vi "Gui_SetupData.vi"(8 "error in (no error)":errorcluster, 11 "Variant":variant) -> (0 "error out":errorcluster caption="sortie d'erreur", 3 "Variant out":variant)   [LabVIEW 2018]
doc: "This VI setup the parameters for the data acquisition.\n\n1. Init the controls with the previous values.\n2. Wait for the user events, CTRL-Z is disabled.\n3. If Acquisition Duration, Record Length or Sample Rate vaues are changed, update the other controls accordingly.\n4. Limit the Record Length value to 32000000, as this is the max memory size of the board."
uses:
  controls/DATA_Inputs.ctl
  controls/SEQUENCE_Inputs.ctl
  controls/EXCIT_Inputs.ctl
  controls/TIMING_Inputs.ctl
  controls/PROCESSING_Inputs.ctl
  controls/TRAPPING_Inputs.ctl
panel:
  in  "CANCEL":bool
  in  "Vertical Range (pk-pk)":dbl(ring)=10.0 caption="Sample Rate" items=["0.2"=0.2, "0.4"=0.4, "1"=1.0, "2"=2.0, "4"=4.0, "10"=10.0]
  in  "OK":bool
  out "Number Of Acquisitions":i16
  out "DATA Inputs":T1={"Record Length"=100000, "Sample Rate"=10000000.0, "Data Type"=0, "Vertical Range"=10.0, "Acquisition Duration"=100000.0} {"Vertical Range" items=["0.2"=0.2, "0.4"=0.4, "1"=1.0, "2"=2.0, "4"=4.0, "10"=10.0]; "Data Type" items=["I16", "DBL"]; "Sample Rate" items=["1 MHz"=1000000.0, "2 MHz"=2000000.0, "5 MHz"=5000000.0, "10 MHz"=10000000.0, "20 MHz"=20000000.0, "25 MHz"=25000000.0, "50 MHz"=50000000.0, "100 MHz"=100000000.0]}
  in  "Sample Rate":dbl(ring)=10000000.0 items=["1 MHz"=1000000.0, "2 MHz"=2000000.0, "5 MHz"=5000000.0, "10 MHz"=10000000.0, "20 MHz"=20000000.0, "25 MHz"=25000000.0, "50 MHz"=50000000.0, "100 MHz"=100000000.0]
  in  "Acquisition Duration (ms)":dbl
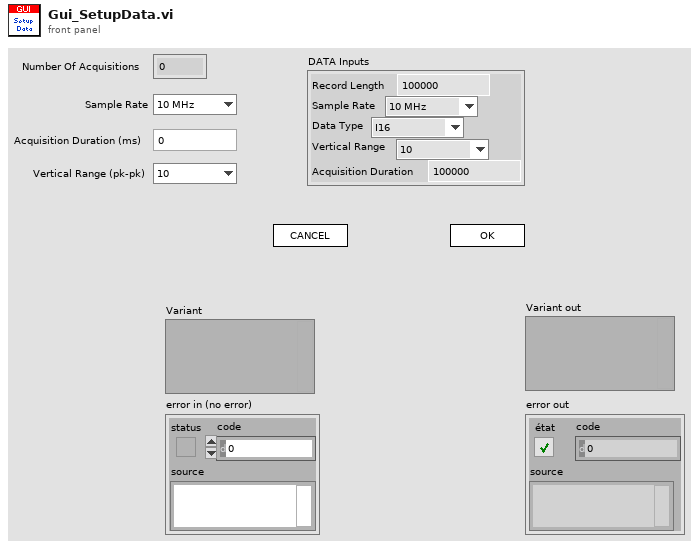
[diagram p1: front panel]
types:
  T1 = typedef "DATA_Inputs.ctl" = cluster{"Record Length":i32, "Sample Rate":dbl, "Data Type":u8, "Vertical Range":dbl, "Acquisition Duration":dbl}
  T2 = typedef "SEQUENCE_Inputs.ctl" = cluster{"EXCIT Inputs":T3, "DATA Inputs":T1, "TIMING Inputs":T4, "PROCESSING Inputs":T5, "TRAPPING Inputs":T6}
  T3 = typedef "EXCIT_Inputs.ctl" = cluster{"Number of Excitations":i32, "Script Text":string, "Table of Waveforms":string[]}
  T4 = typedef "TIMING_Inputs.ctl" = cluster{"Number of Acquisitions ":i16, "Number of Accumulations":i16, "Table of Waveforms":string[], "Script Text":string}
  T5 = typedef "PROCESSING_Inputs.ctl" = cluster{"Reference Mass":dbl, "Cyclotron Freq":dbl, "Magnetron Freq":dbl}
  T6 = typedef "TRAPPING_Inputs.ctl" = cluster{"Number of Channels":i32, "Init Values":dbl[], "Opening Values":dbl[], "Trapping Values":dbl[], "Emptying Values":dbl[], "Adiabatic ON":bool, "Adiabatic Duration":i32, "Adiabatic Waveforms":string[], "Ions Refill ON":bool, "Number of Ions Refills":i32, "Trapping Delay":dbl, "Trapping Duration":dbl}
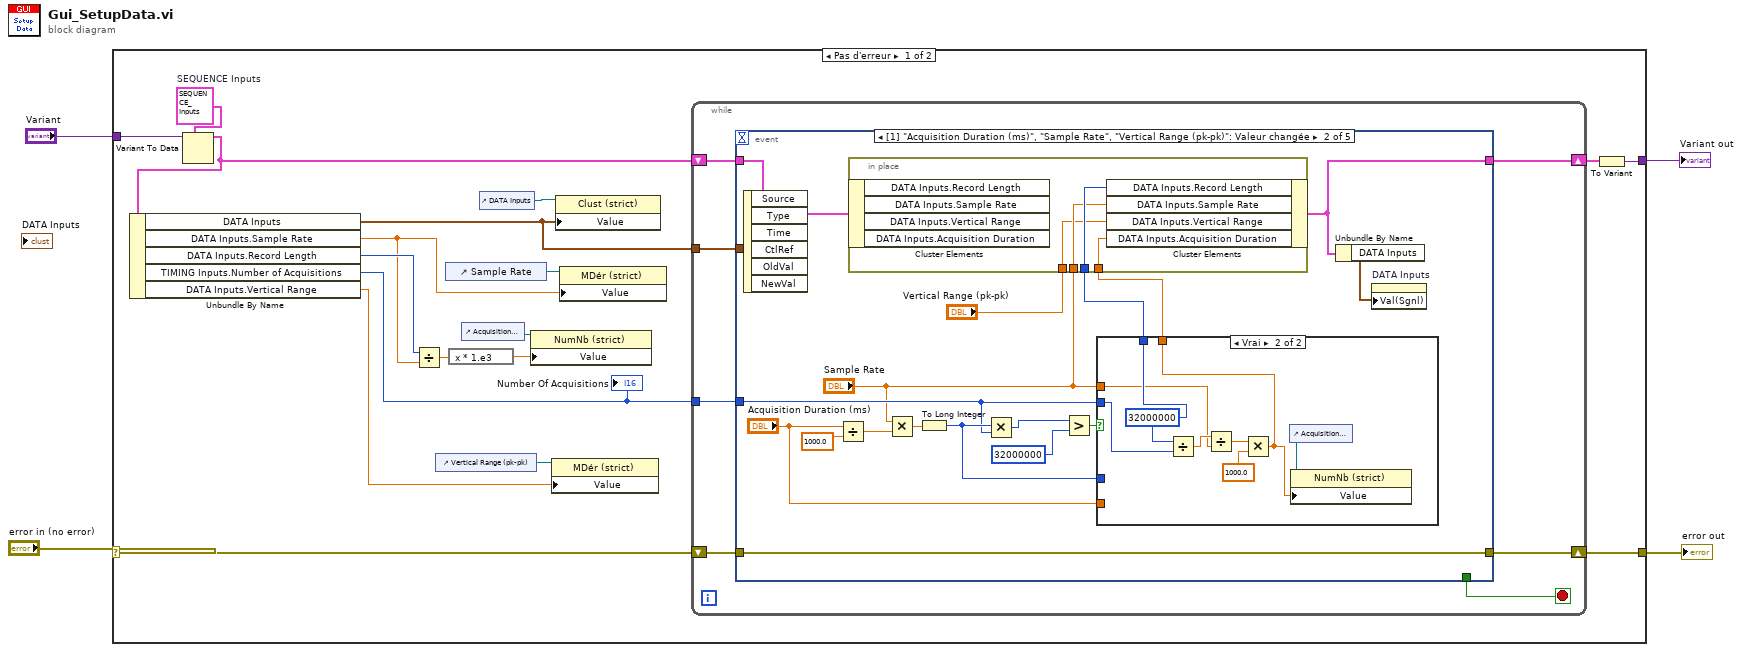
[diagram p0: block diagram]
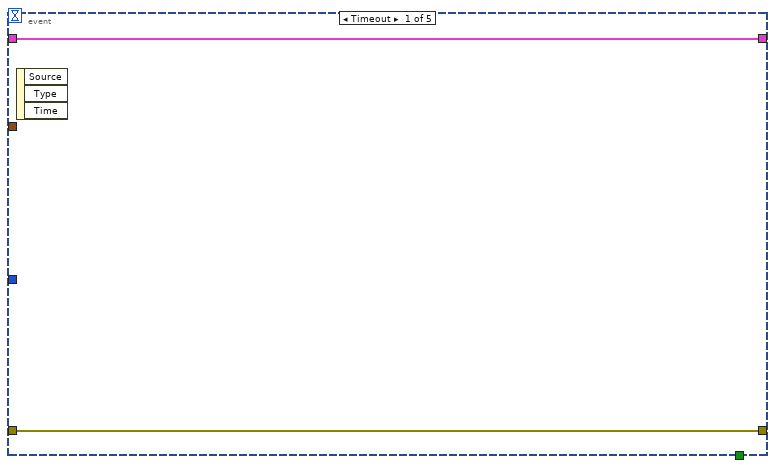
[diagram p2: hidden frame]
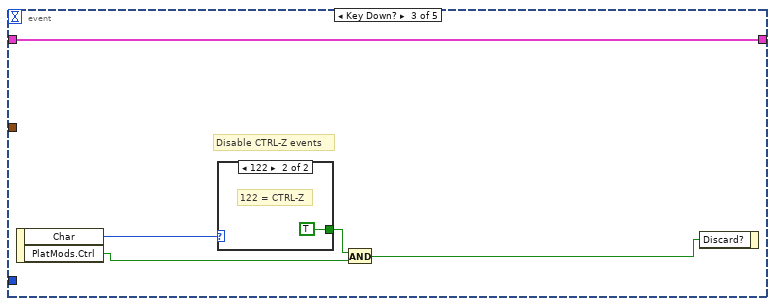
[diagram p4: hidden frame]
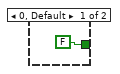
[diagram p5: hidden frame]
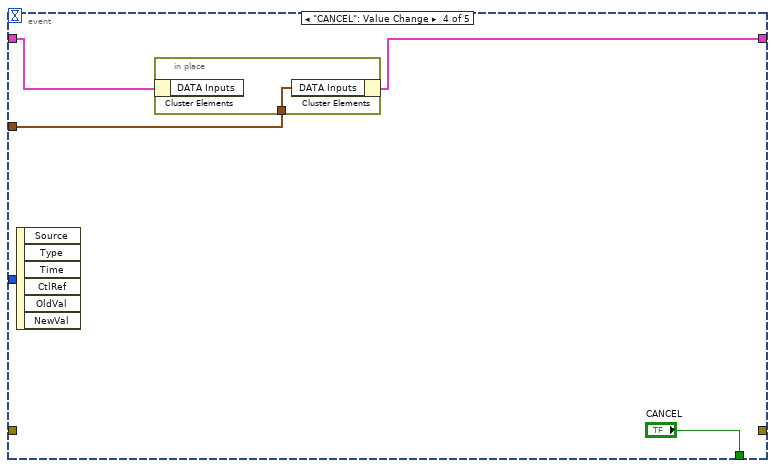
[diagram p6: hidden frame]
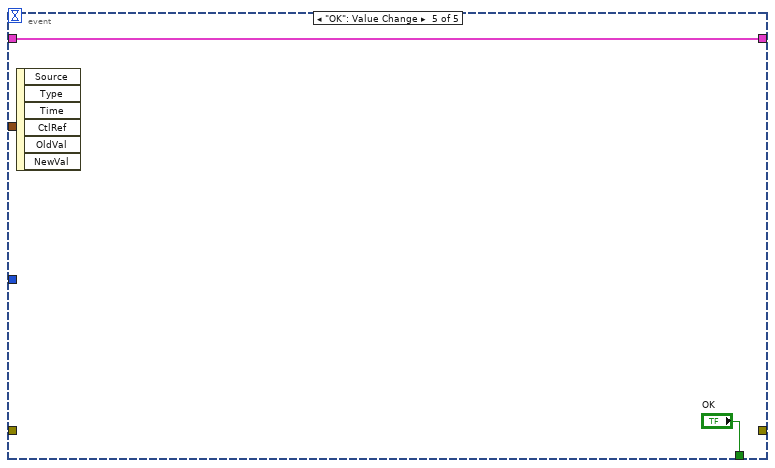
[diagram p7: hidden frame]
diagram:
  n1 = case shown="Pas d'erreur" "error in (no error)" {
    selector: "error in (no error)" -> [w22 w78]
    tunnel: [w21 w78] -> w3
    tunnel: "Variant" -> [w19 w77]
    tunnel: [w10 w77] -> w1
    frame No Error {
      w20 = T2 {"EXCIT Inputs"={"Number of Excitations"=1, "Script Text"="", "Table of Waveforms"=[]}, "DATA Inputs"={"Record Length"=8192, "Sample Rate"=4.0, "Data Type"=0, "Vertical Range"=0.0, "Acquisition Duration"=100000.0}, "TIMING Inputs"={"Number of Acquisitions "=1, "Number of Accumulations"=1, "Table of Waveforms"=[], "Script Text"=""}, "PROCESSING Inputs"={"Reference Mass"=300.0939, "Cyclotron Freq"=255.727, "Magnetron Freq"=0.001}, "TRAPPING Inputs"={"Number of Channels"=4, "Init Values"=[2.0, 5.0, 5.0, 2.0], "Opening Values"=[0.0, 0.0, 0.0, 0.0], "Trapping Values"=[2.0, 5.0, 5.0, 2.0], "Emptying Values"=[-5.0, -5.0, -5.0, -5.0], "Adiabatic ON"=FALSE, "Adiabatic Duration"=0, "Adiabatic Waveforms"=["Adiabatic_None_2_2_2000.bin", "Adiabatic_Ramp_5_0_2000.bin", "Adiabatic_DoubleRamp_5_0_2000.bin", "Adiabatic_RC_2_0_2000.bin"], "Ions Refill ON"=FALSE, "Number of Ions Refills"=4, "Trapping Delay"=400.0, "Trapping Duration"=300.0}}  # SEQUENCE Inputs
      n2 = Variant To Data(type=w20, Variant=w19) -> (data=w18:T2)  [unwired: 1 in, 1 out]
      n3 = Unbundle By Name(w18) -> ("DATA Inputs"=w5:T1, "DATA Inputs.Sample Rate"=w13:dbl, "DATA Inputs.Record Length"=w15:i32, "TIMING Inputs.Number of Acquisitions"=w8:i16, "DATA Inputs.Vertical Range"=w6:dbl)
      "Number Of Acquisitions" <- w8
      n4 = Divide(x=w15, y=w13) -> (x/y=w14:dbl)
      n5 = control-ref of="Vertical Range (pk-pk)"() -> (w7:refnum<vi>)
      n6 = control-ref of="Sample Rate"() -> (w17:refnum<vi>)
      n7 = expression code="x * 1.e3"(w14) -> (w16:dbl)
      n8 = control-ref of="Acquisition Duration (ms)"() -> (w12:refnum<vi>)
      n9 = control-ref of="DATA Inputs"() -> (w9:refnum<vi>)
      n10 = property class="NumNb (strict)"(reference=w12, "Value"=w16) -> ()  [unwired: 1 in, 2 out]
      n11 = property class="MDér (strict)"(reference=w7, "Value"=w6) -> ()  [unwired: 1 in, 2 out]
      n12 = property class="Clust (strict)"(reference=w9, "Value"=w5) -> ()  [unwired: 1 in, 2 out]
      n13 = property class="MDér (strict)"(reference=w17, "Value"=w13) -> ()  [unwired: 1 in, 2 out]
      n14 = while {
        shift-right: [w25] -> w21
        shift-left: w22 -> [w26]
        shift-right: [w27] -> w11
        shift-left: w18 -> [w29]
        tunnel: w8 -> [w28]
        tunnel: w5 -> [w23]
        stop <- w24 stop-if-true
        n15 = event shown="[1] \"Acquisition Duration (ms)\", \"Sample Rate\", \"Vertical Range (pk-pk)\": Valeur changée" {
          selector: _ -> [_ _ _ _ _]
          dyn-events: _ -> [_ _ _ _ _]
          timeout: _ -> [_ _ _ _ _]
          tunnel: w29 -> [w31 w48 w63 w73 w75]
          tunnel: w28 -> [_ w41 _ _ _]
          tunnel: [w31 w33 w63 w72 w75] -> w27
          tunnel: w26 -> [w30 w34 _ _ _]
          tunnel: [w30 w34 _ _ _] -> w25
          tunnel: [_ _ _ "CANCEL" "OK"] -> w24
          tunnel: w23 -> [_ _ _ w71 _]
          event Timeout {
            n16 = event-data() -> ()  [unwired: 1 in, 3 out]
          }
          event "Acquisition Duration (ms)", "Sample Rate", "Vertical Range (pk-pk)": Value Change {
            n17 = event-data() -> ()  [unwired: 1 in, 6 out]
            n18 = Divide(x="Acquisition Duration (ms)", y=1000.0) -> (x/y=w47:dbl)
            n19 = Multiply(x="Sample Rate", y=w47) -> (x*y=w46:dbl)
            n20 = To Long Integer(number=w46) -> (32bit integer=w42:i32)
            n21 = Multiply(x=w42, y=w41) -> (x*y=w44:i32)
            n22 = Greater?(x=w44, y=32000000) -> (0:w45:bool)
            n23 = case shown="Vrai" w45 {
              tunnel: "Sample Rate" -> [_ w57]
              tunnel: w41 -> [_ w62]
              tunnel: [w54 w58] -> w40
              tunnel: w42 -> [w54 _]
              tunnel: "Acquisition Duration (ms)" -> [w53 _]
              tunnel: [w53 w55] -> w35
              frame False {
              }
              frame True {
                w58 = 32000000 ("x")
                n24 = Divide(x=w58, y=w62) -> (x/y=w61:dbl)
                n25 = Divide(x=w61, y=w57) -> (x/y=w60:dbl)
                n26 = Multiply(x=w60, y=1000.0) -> (x*y=w55:dbl)
                n27 = control-ref of="Acquisition Duration (ms)"() -> (w56:refnum<vi>)
                n28 = property class="NumNb (strict)"(reference=w56, "Value"=w55) -> ()  [unwired: 1 in, 2 out]
              }
            }
            n29 = in-place {
              in-place-border: w40 -> [w52]
              in-place-border: "Sample Rate" -> [w51]
              in-place-border: "Vertical Range (pk-pk)" -> [w50]
              in-place-border: w35 -> [w49]
              n30 = in-place-cluster #1(w48) -> ()  [unwired: 4 out]
              n31 = in-place-cluster #1("DATA Inputs.Record Length"=w52, "DATA Inputs.Sample Rate"=w51, "DATA Inputs.Vertical Range"=w50, "DATA Inputs.Acquisition Duration"=w49) -> (w33:T2)
            }
            n32 = Unbundle By Name(w33) -> ("DATA Inputs"=w32:T1)
            n33 = property on="DATA Inputs" class="Clust (strict)"("Val(Sgnl)"=w32) -> ()  [unwired: 2 in, 2 out]
          }
          event Key Down? {
            # "Disable CTRL-Z events"
            n34 = event-data() -> ("Char"=w66:i16, "PlatMods.Ctrl"=w65:bool)  [unwired: 1 in]
            n35 = case shown="122" w66 {
              tunnel: [FALSE TRUE] -> w67
              frame 0, Default {
              }
              frame 122 {
                # "122 = CTRL-Z"
              }
            }
            n36 = And(x=w67, y=w65) -> (x .and. y?=w64:bool)
            n37 = event-data("Discard?"=w64) -> ()  [unwired: 1 in, 1 out]
          }
          event "CANCEL": Value Change {
            n38 = event-data() -> ()  [unwired: 1 in, 6 out]
            n39 = in-place {
              in-place-border: w71 -> [w74]
              n40 = in-place-cluster #2(w73) -> ()  [unwired: 1 out]
              n41 = in-place-cluster #2("DATA Inputs"=w74) -> (w72:T2)
            }
          }
          event "OK": Value Change {
            n42 = event-data() -> ()  [unwired: 1 in, 6 out]
          }
        }
      }
      n43 = To Variant(anything=w11) -> (Variant=w10:variant)
    }
    frame Error {
    }
  }
  "error out" <- w3
  "Variant out" <- w1
